vi "Process.vi"(8 "error in":errorcluster, 11 "SMO.ByRefWithEvents":refnum<class "SMO.ByRefWithEvents.lvclass">) -> (0 "error out":errorcluster, 3 "SMO.ByRefWithEvents out":refnum<class "SMO.ByRefWithEvents.lvclass">)   [LabVIEW 2013, in "SMO.ByRefWithEvents.lvclass"]
doc: "---------------------------------------------------------------\nJKI State Machine Objects™\nhttp://jki.net/state-machine-objects/\nCopyright (C) 2005-2015, JKI <info@jki.net>\nALL RIGHTS RESERVEDJKI State Machine Objects (SMO) 1.0.0.5\nJKI - JKI\nCopyright (c) 2016, JKI"
uses:
  SMO.ByRefWithEvents.lvclass
  <vilib>/JKI/JKI SMO/SMO/Typedefs/Parent Call--Enum.ctl
  <vilib>/JKI/JKI SMO/SMO/SMO.lvclass
panel:
  # "For instructions on how to use the JKI State Machine Objects, examples and video tutorials, visit:\nhttp://jki.net/state-machine-objects/\n\nJKI State Machine Objects™\nhttp://jki.net/state-machine-objects/\nCopyright (C) 2005-2015, JKI <info@jki.net>\nALL RIGHTS RESERVED"
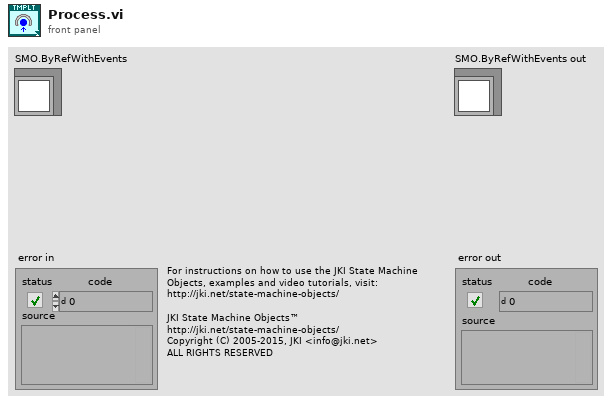
[diagram p1: front panel]
types:
  T1 = typedef "SMO.lvclass/Parent Call--Enum.ctl" = enum16{"Allows parent to run", "Does not request parent to run"}
  T2 = enum32{"invalid app kind", "Development System", "Run Time System", "Student Edition", "Embedded LabVIEW", "Evaluation", "Custom"}
  T3 = enum32{"Invalid", "Standard", "Closed", "Hidden", "Minimized", "Maximized"}
  T4 = enum32{"Bad", "Idle", "Run top level", "Running"}
  T5 = cluster{"Core":cluster{"Current VI Reference":refnum<vi>, "Close Panel on Exit?":bool, "error":errorcluster}, "Self Reference":refnum<class "SMO.ByRefWithEvents.lvclass">, "Your string data":string}
  T6 = cluster{"Current VI Reference":refnum<vi>, "Close Panel on Exit?":bool, "error":errorcluster}
  T7 = typedef "SMO.lvclass/Protected Events.ctl" = cluster{"StopProcesses":refnum<user-event>, "AbortProcesses":refnum<user-event>}
  T8 = typedef "SMO.ByRefWithEvents.lvclass/ProtectedEvents--Cluster.ctl" = cluster{"API_Template":refnum<user-event>}
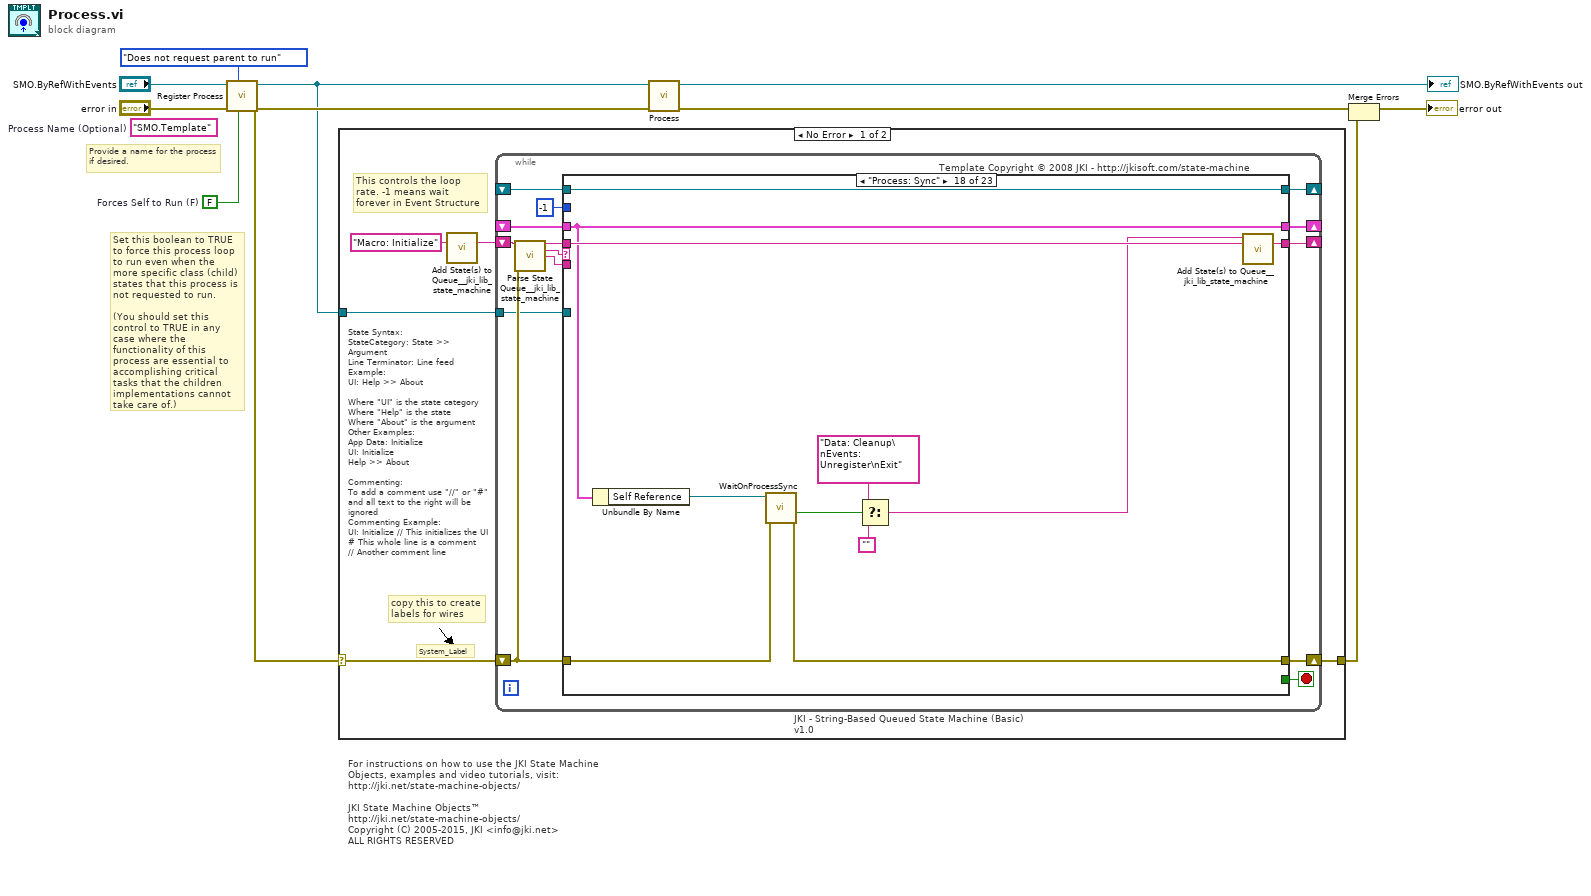
[diagram p0: block diagram]
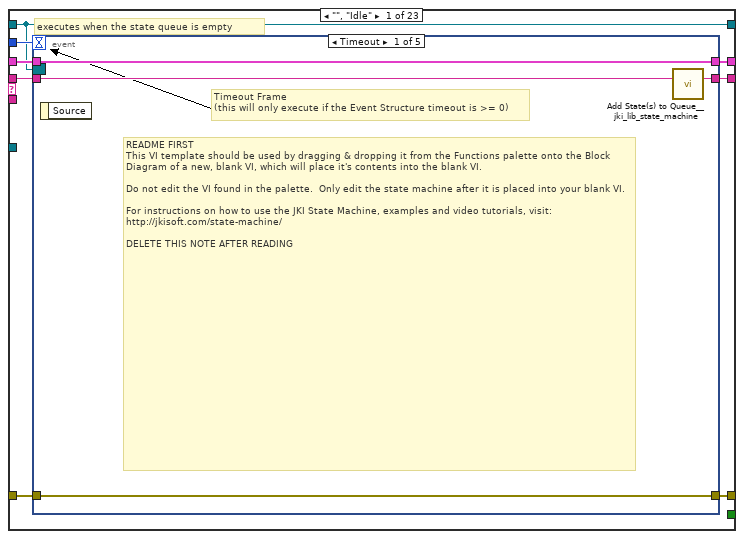
[diagram p2: hidden frame]
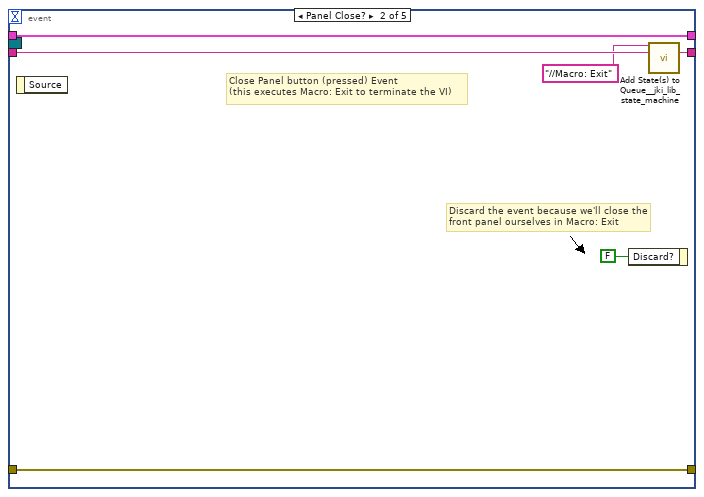
[diagram p3: hidden frame]
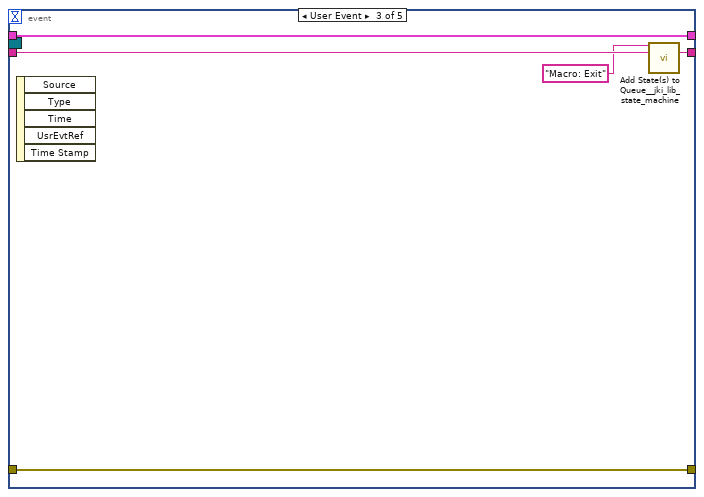
[diagram p4: hidden frame]
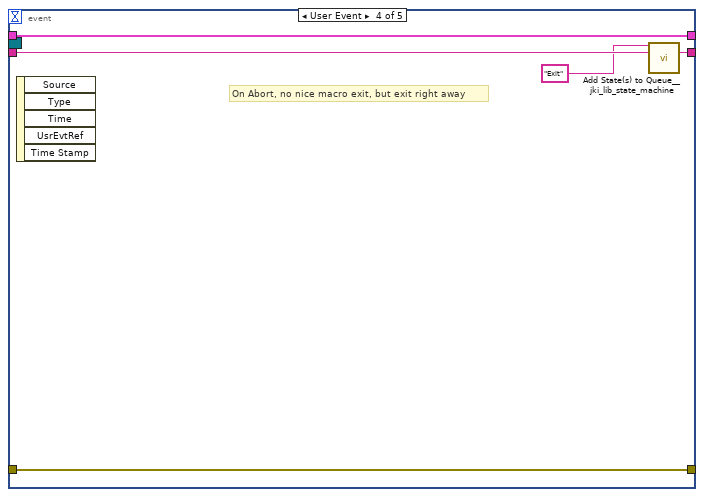
[diagram p5: hidden frame]
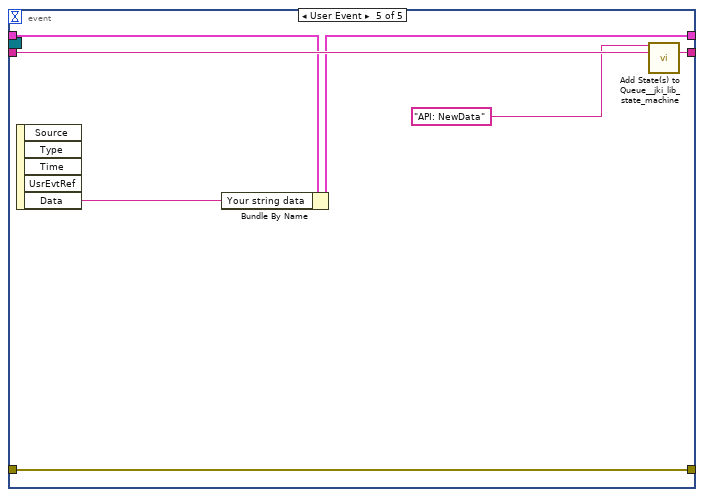
[diagram p6: hidden frame]
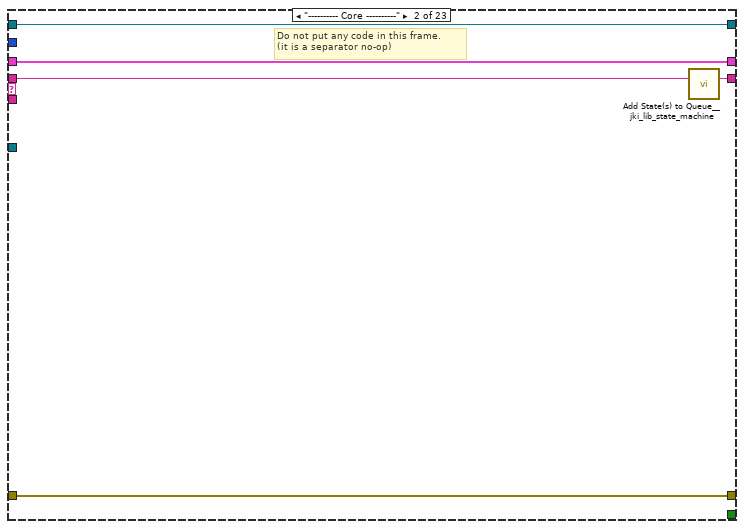
[diagram p7: hidden frame]
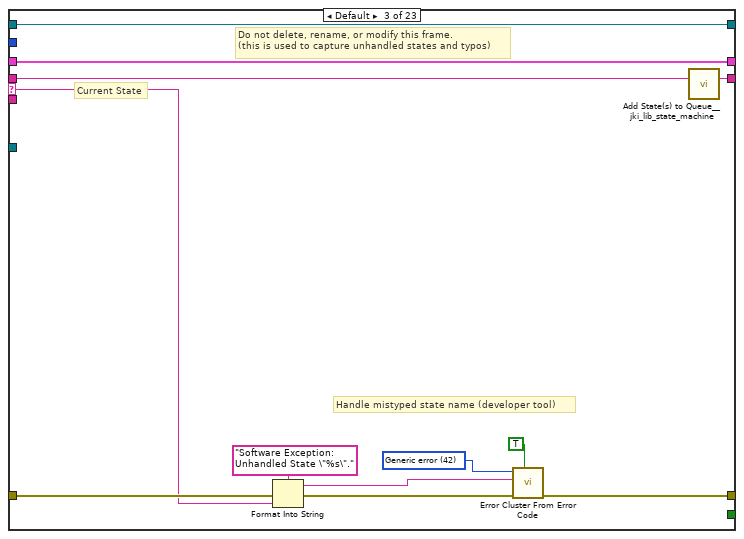
[diagram p8: hidden frame]
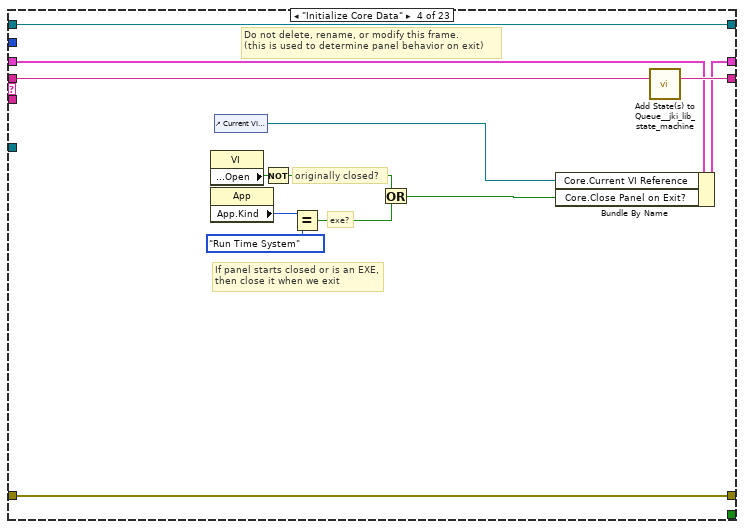
[diagram p9: hidden frame]
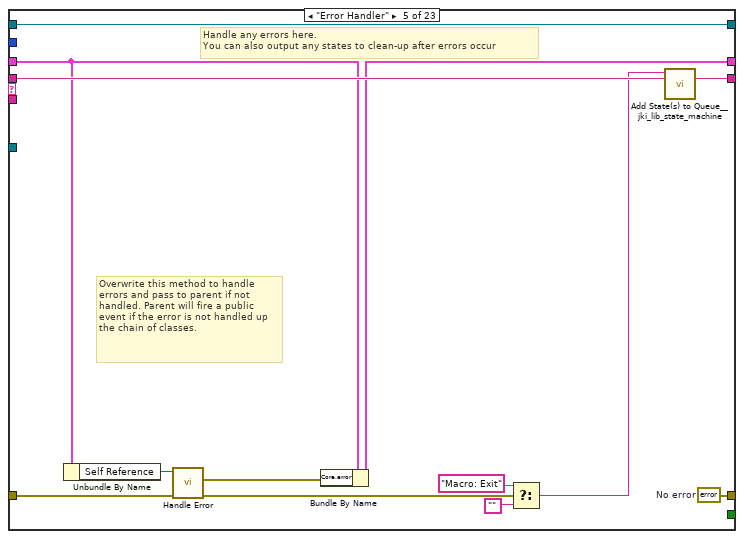
[diagram p10: hidden frame]
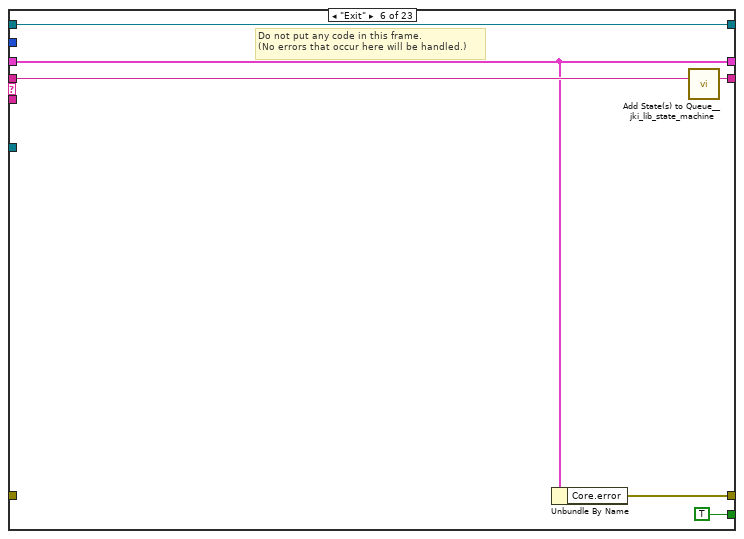
[diagram p11: hidden frame]
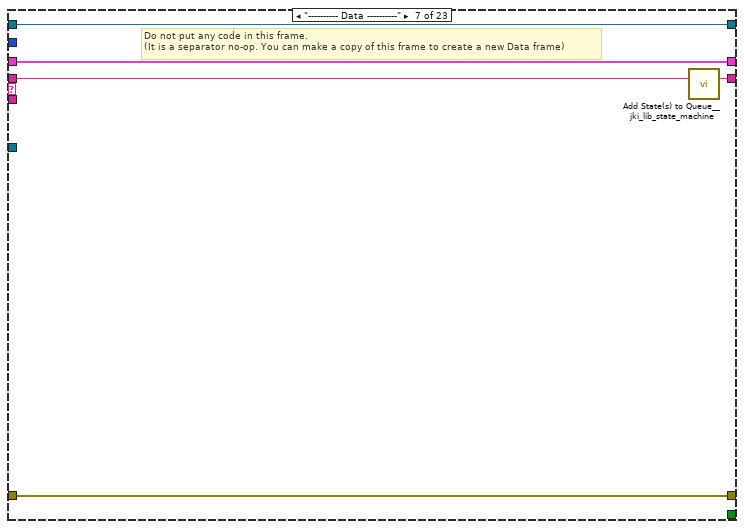
[diagram p12: hidden frame]
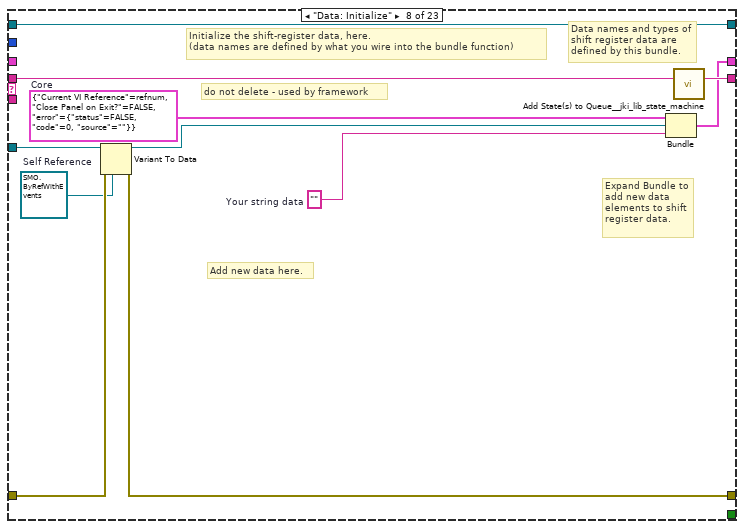
[diagram p13: hidden frame]
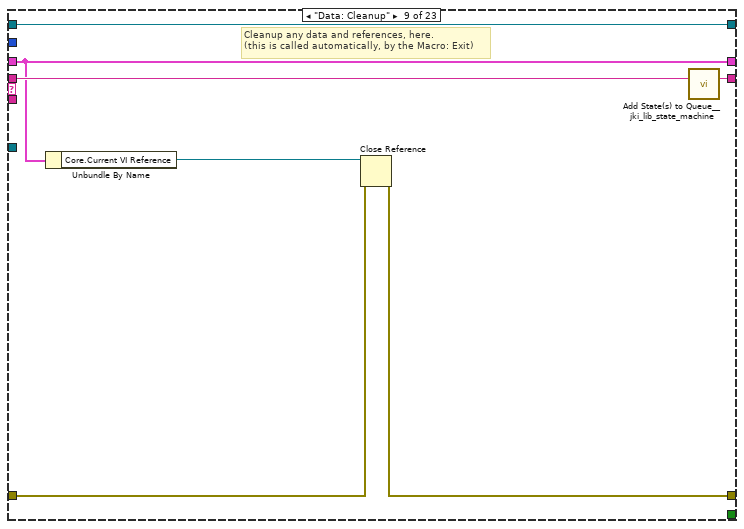
[diagram p14: hidden frame]
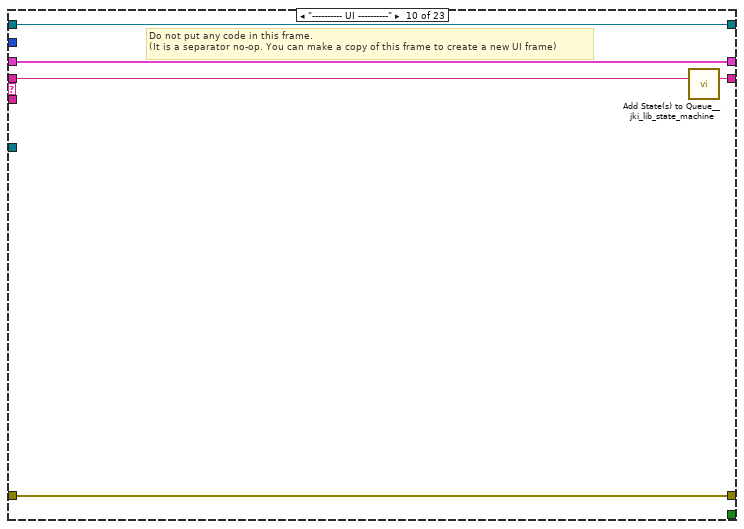
[diagram p15: hidden frame]
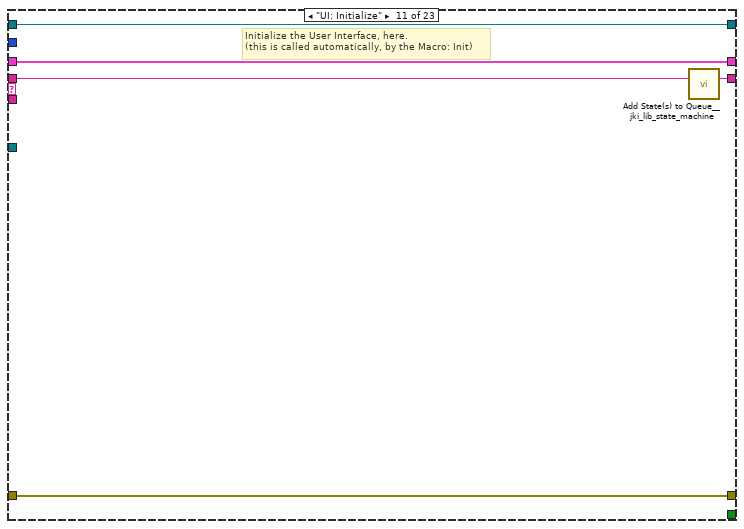
[diagram p16: hidden frame]
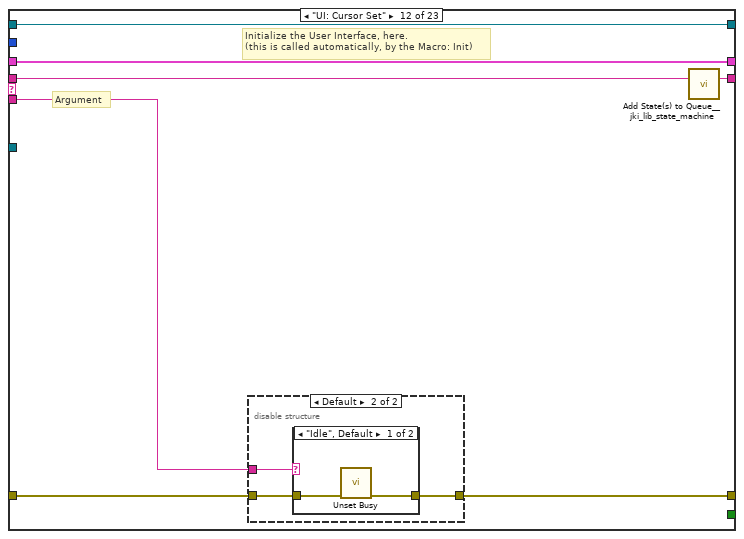
[diagram p17: hidden frame]
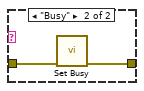
[diagram p19: hidden frame]
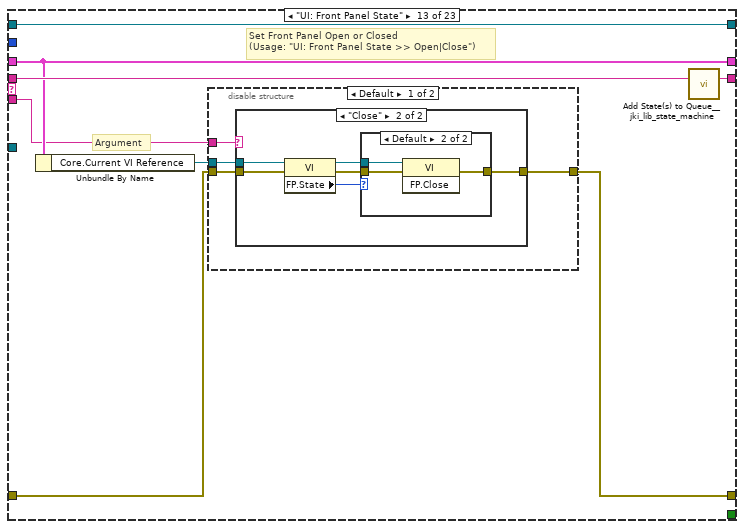
[diagram p20: hidden frame]
diagram:
  w1 = FALSE  # Forces Self to Run (F)
  (unwired) "SMO.Template"  # Process Name (Optional)
  # "Provide a name for the process\nif desired."
  # "Set this boolean to TRUE to force this process loop to run even when the more specific class (child) states that this process is not requested to run.\n\n(You should set this control to TRUE in any case where the functionality of this process are essential to accomplishing critical tasks that the children implementations cannot take care of.)"
  # "For instructions on how to use the JKI State Machine Objects, examples and video tutorials, visit:\nhttp://jki.net/state-machine-objects/\n\nJKI State Machine Objects™\nhttp://jki.net/state-machine-objects/\nCopyright (C) 2005-2015, JKI <info@jki.net>\nALL RIGHTS RESERVED"
  n1 = call <vilib>:"Register Process.vi"("Forces Self to Run (F)"=w1, "Parent Call"=Parent_Call--Enum."Does not request parent to run", "error in (no error)"="error in", "SMO"="SMO.ByRefWithEvents") -> ("error out"=w7:errorcluster, "SMO out"=w6:refnum<class "SMO.ByRefWithEvents.lvclass">)  [unwired: 6 in]
  n2 = case shown="No Error" w7 {
    selector: w7 -> [w12 w295]
    tunnel: w6 -> [w13 _]
    tunnel: [w11 w295] -> w3
    frame No Error {
      # "State Syntax:\nStateCategory: State >> Argument\nLine Terminator: Line feed\nExample:\nUI: Help >> About\n\nWhere \"UI\" is the state category\nWhere \"Help\" is the state\nWhere \"About\" is the argument\nOther Examples:\nApp Data: Initialize\nUI: Initialize\nHelp >> About\n\nCommenting:\nTo add a comment use \"//\" or \"#\" and all text to the right will be ignored\nCommenting Example:\nUI: Initialize // This initializes the UI\n# This whole line is a comment\n// Another comment line"
      # "copy this to create labels for wires"
      # "This controls the loop rate. -1 means wait forever in Event Structure"
      # "System_Label"
      n3 = call <vilib>:"Add State(s) to Queue__jki_lib_state_machine.vi"("State(s) in (\"\")"="Macro: Initialize") -> ("States Out"=w15:string)  [unwired: 14 in]
      n4 = while "JKI - String-Based Queued State Machine (Basic) v1.0" {
        shift-right: [w22] -> _
        shift-left: _ -> [w21]
        shift-right: [w25] -> w11
        shift-left: w12 -> [w19]
        shift-right: [w24] -> _
        shift-left: w15 -> [w26]
        tunnel: w13 -> [w18]
        shift-right: [w17] -> _
        shift-left: _ -> [w16]
        stop <- w23 stop-if-true
        # "Template Copyright © 2008 JKI - http://jkisoft.com/state-machine"
        n5 = call <vilib>:"Parse State Queue__jki_lib_state_machine.vi"("State Queue"=w26, "Error In (no error)"=w19) -> ("Remaining States"=w28:string, "Current State"=w29:string, "Arguments"=w27:string)  [unwired: 11 in]
        n6 = case shown="\"Process: Sync\"" w29 {
          selector: w29 -> [_ _ w71 _ _ _ _ _ _ _ _ _ _ _ _ _ _ _ _ _ _ _ _]
          tunnel: w28 -> [w37 w69 w75 w94 w107 w113 w118 w129 w136 w141 w146 w153 w169 w201 w215 w229 w234 w245 w250 w264 w281 w286 w294]
          tunnel: w27 -> [_ _ _ _ _ _ _ _ _ _ _ w147 w163 _ _ _ _ _ _ _ _ _ _]
          tunnel: w21 -> [w35 w66 w73 w85 w96 w109 w115 _ w131 w138 w144 w151 w165 w198 w211 w220 w231 w242 w247 w262 w279 w284 w291]
          tunnel: [w34 w67 w77 w91 w98 w108 w116 w124 w132 w139 w143 w148 w166 w199 w213 w227 w232 w236 w248 w260 w276 w282 w287] -> w25
          tunnel: w19 -> [w33 w67 w76 w91 w103 _ w116 w125 w133 w139 w143 w149 w167 w199 w213 w227 w232 w237 w248 w261 w277 w282 w288]
          tunnel: [w36 w68 w74 w93 w106 w112 w117 w128 w135 w140 w145 w152 w168 w200 w214 w228 w233 w244 w249 w263 w280 w285 w293] -> w24
          tunnel: [_ _ _ _ _ TRUE _ _ _ _ _ _ _ _ _ _ _ _ _ _ _ _ _] -> w23
          tunnel: [w32 w66 w73 w92 w95 w109 w115 w127 w131 w138 w144 w151 w165 w198 w211 w220 w231 w242 w247 w262 w279 w284 w291] -> w22
          tunnel: -1 ("Timeout") -> [w31 _ _ _ _ _ _ _ _ _ _ _ _ _ _ _ _ _ _ _ _ _ _]
          tunnel: w18 -> [_ _ _ _ _ _ _ w122 _ _ _ _ _ _ _ _ _ _ _ _ _ _ _]
          tunnel: [w30 w65 w70 w82 w105 w110 w114 w120 w130 w137 w142 w150 w162 w197 w212 w221 w230 w243 w246 w259 w278 w283 w292] -> w17
          tunnel: w16 -> [w30 w65 w70 w82 w105 w110 w114 w120 w130 w137 w142 w150 w162 w197 w212 w221 w230 w243 w246 w251 w278 w283 w292]
          frame "", "Idle" {
            # "executes when the state queue is empty"
            n7 = event shown="[0] Timeout" {
              selector: w30 -> [_ _ _ _ _]
              dyn-events: _ -> [_ _ _ _ _]
              timeout: w31 -> [_ _ _ _ _]
              tunnel: w37 -> [w41 w47 w52 w57 w64]
              tunnel: [w40 w46 w51 w56 w63] -> w36
              tunnel: w35 -> [w38 w44 w49 w54 w60]
              tunnel: [w39 w45 w50 w55 w62] -> w34
              tunnel: w33 -> [w39 w45 w50 w55 w62]
              tunnel: [w38 w44 w49 w54 w59] -> w32
              event Timeout {
                # "README FIRST\nThis VI template should be used by dragging & dropping it from the Functions palette onto the Block Diagram of a new, blank VI, which will place it's contents into the blank VI.\n\nDo not edit the VI found in the palette.  Only edit the state machine after it is placed into your blank VI.\n\nFor instructions on how to use the JKI State Machine, examples and video tutorials, visit:\nhttp://jkisoft.com/state-machine/\n\nDELETE THIS NOTE AFTER READING"
                # "Timeout Frame\n(this will only execute if the Event Structure timeout is >= 0)"
                n8 = event-data() -> ()  [unwired: 1 in, 1 out]
                n9 = call <vilib>:"Add State(s) to Queue__jki_lib_state_machine.vi"("State(s) in (\"\")"=w41) -> ("States Out"=w40:string)  [unwired: 14 in]
              }
              event Panel Close? {
                # "Discard the event because we'll close the front panel ourselves in Macro: Exit"
                # "Close Panel button (pressed) Event\n(this executes Macro: Exit to terminate the VI)"
                n10 = event-data() -> ()  [unwired: 1 in, 1 out]
                n11 = event-data("Discard?"=FALSE) -> ()  [unwired: 1 in, 1 out]
                n12 = call <vilib>:"Add State(s) to Queue__jki_lib_state_machine.vi"("State(s) in Front (\"\")"="//Macro: Exit", "State(s) in (\"\")"=w47) -> ("States Out"=w46:string)  [unwired: 13 in]
              }
              event User Event {
                n13 = event-data() -> ()  [unwired: 1 in, 5 out]
                n14 = call <vilib>:"Add State(s) to Queue__jki_lib_state_machine.vi"("State(s) in Front (\"\")"="Macro: Exit", "State(s) in (\"\")"=w52) -> ("States Out"=w51:string)  [unwired: 13 in]
              }
              event User Event {
                # "On Abort, no nice macro exit, but exit right away"
                n15 = event-data() -> ()  [unwired: 1 in, 5 out]
                n16 = call <vilib>:"Add State(s) to Queue__jki_lib_state_machine.vi"("State(s) in Front (\"\")"="Exit", "State(s) in (\"\")"=w57) -> ("States Out"=w56:string)  [unwired: 13 in]
              }
              event User Event {
                n17 = event-data() -> ("Data"=w61:string)  [unwired: 1 in, 4 out]
                n18 = Bundle By Name(cluster=w60, "Your string data"=w61) -> (w59:T5)
                n19 = call <vilib>:"Add State(s) to Queue__jki_lib_state_machine.vi"("State(s) in Front (\"\")"="API: NewData", "State(s) in (\"\")"=w64) -> ("States Out"=w63:string)  [unwired: 13 in]
              }
            }
          }
          frame "---------- Core ----------" {
            # "Do not put any code in this frame.\n(it is a separator no-op)"
            n20 = call <vilib>:"Add State(s) to Queue__jki_lib_state_machine.vi"("State(s) in (\"\")"=w69) -> ("States Out"=w68:string)  [unwired: 14 in]
          }
          frame Default {
            w80 = 42 items=["No error", "Argument error", "Memory is full", "Out of zone", "End of file", "File already open", "Generic file I/O error", "File not found", "File permission error", "Disk is full", "Duplicate path", "Too many files open", "System feature not enabled", "Resource file not found", "Cannot add resource", "Resource not found", "Image not found", "Image memory error", "Pen does not exist", "Config type invalid", "Config token not found", "Config parse error", "Config memory error", "Bad external code format", "Bad external code offset", "External code not present", "Null window", "Destroy window error", "Null menu", "Print aborted", "Bad print record", "Print driver error", "Windows error during printing", "Memory error during printing", "Print dialog error", "Generic print error", "Invalid device refnum", "Device not found", "Device parameter error", "Device unit error", "Cannot open device", "Device call aborted", "Generic error", "Cancelled by user", "Object ID too low", "Object ID too high", "Object not in heap", "Unknown heap", "Unknown object (invalid DefProc)", "Unknown object (DefProc not in table)", "Message out of range", "Invalid (null) method", "Unknown message", "Manager call not supported", "Bad address", "Network operation in progress", "Network operation timed out", "Connection is busy", "Network attribute not supported", "Network error", "Address in use", "System out of memory", "Connection aborted", "Connection refused", "Not connected", "Already connected", "Connection closed", "Initialization error (interapplication manager)", "Bad occurrence", "Wait on unbound occurrence handler", "Occurrence queue overflow", "Datalog type conflict", "Unused", "Unrecognized type (interapplication manager)", "Memory corrupt", "Failed to make temporary DLL", "Old CIN version", "Drag socket not found", "Failed to load drop-object", "Failed to register OLE object", "Failed to release OLE object", "Format specifier type mismatch", "Unknown format specifier", "Too few format specifiers", "Too many format specifiers", "Scan failed", "Newer CIN version", "Error converting to variant", "Runtime menu error", "Password tampered", "Variant attribute not found", "Incompatible variant data type", "Event data is not available", "Event Store is not present", "Occurrence is not found", "Event Queue is not created", "Event info is not available", "Refnum passed is NULL", "Error retrieving Class GUID", "Error retrieving CoClass GUID", "Error retrieving TypeLib GUID.", "Bad built application magic bytes.", "Specific driver is different from the specific driver associated with the Logical Name.", "There is no session opened to the class driver.", "Max Error", "MAX - Error with config objects", "MAX - Error loading configuration", "MAX - Group not supported"]
            # "Current State"
            # "Do not delete, rename, or modify this frame.\n(this is used to capture unhandled states and typos)"
            # "Handle mistyped state name (developer tool)"
            n21 = Format Into String(format string="Software Exception: Unhandled State \"%s\"." ("message"), error in=w76, w71) -> (resulting string=w79:string, error out=w78:errorcluster)  [unwired: 1 in]
            n22 = call <vilib>:"Error Cluster From Error Code.vi"("show call chain? (False)"=TRUE, "error in (no error)"=w78, "error message (\"\")"=w79, "error code (0)"=w80) -> ("error out"=w77:errorcluster)  [unwired: 5 in]
            n23 = call <vilib>:"Add State(s) to Queue__jki_lib_state_machine.vi"("State(s) in (\"\")"=w75) -> ("States Out"=w74:string)  [unwired: 14 in]
          }
          frame "Initialize Core Data" {
            # "Do not delete, rename, or modify this frame.\n(this is used to determine panel behavior on exit)"
            # "originally closed?"
            # "exe?"
            # "If panel starts closed or is an EXE, then close it when we exit"
            n24 = property class="VI"() -> ("Front Panel.Open"=w90:bool)  [unwired: 2 in, 2 out]
            n25 = property class="App"() -> ("App.Kind"=w89:T2)  [unwired: 2 in, 2 out]
            n26 = control-ref of="Current VI Reference"() -> (w83:refnum<vi>)
            n27 = Not(x=w90) -> (.not. x?=w87:bool)
            n28 = Equal?(x=w89, y=T2."Run Time System" ("Application:Kind")) -> (x = y?=w86:bool)
            n29 = Or(x=w87, y=w86) -> (x .or. y?=w84:bool)
            n30 = Bundle By Name(cluster=w85, "Core.Current VI Reference"=w83, "Core.Close Panel on Exit?"=w84) -> (w92:T5)
            n31 = call <vilib>:"Add State(s) to Queue__jki_lib_state_machine.vi"("State(s) in (\"\")"=w94) -> ("States Out"=w93:string)  [unwired: 14 in]
          }
          frame "Error Handler" {
            w98 = errorcluster {"status"=FALSE, "code"=0, "source"=""}  # No error
            # "Overwrite this method to handle errors and pass to parent if not handled. Parent will fire a public event if the error is not handled up the chain of classes."
            # "Handle any errors here.\nYou can also output any states to clean-up after errors occur"
            n32 = Unbundle By Name(w96) -> ("Self Reference"=w104:refnum<class "SMO.ByRefWithEvents.lvclass">)
            n33 = call-dynamic "Handle Error.vi"("error in"=w103, "SMO"=w104) -> ("handling error"=w99:errorcluster, "Unhandled error"=w97:errorcluster)  [unwired: 7 in, 1 out]
            n34 = Bundle By Name(cluster=w96, "Core.error"=w97) -> (w95:T5)
            n35 = Select(t="Macro: Exit", s=w99, f="") -> (s? t:f=w100:string)
            n36 = call <vilib>:"Add State(s) to Queue__jki_lib_state_machine.vi"("State(s) in Front (\"\")"=w100, "State(s) in (\"\")"=w107) -> ("States Out"=w106:string)  [unwired: 13 in]
          }
          frame "Exit" {
            # "Do not put any code in this frame.\n(No errors that occur here will be handled.)"
            n37 = Unbundle By Name(w109) -> ("Core.error"=w108:errorcluster)
            n38 = call <vilib>:"Add State(s) to Queue__jki_lib_state_machine.vi"("State(s) in (\"\")"=w113) -> ("States Out"=w112:string)  [unwired: 14 in]
          }
          frame "---------- Data ----------" {
            # "Do not put any code in this frame.\n(It is a separator no-op. You can make a copy of this frame to create a new Data frame)"
            n39 = call <vilib>:"Add State(s) to Queue__jki_lib_state_machine.vi"("State(s) in (\"\")"=w118) -> ("States Out"=w117:string)  [unwired: 14 in]
          }
          frame "Data: Initialize" {
            w119 = T6 {"Current VI Reference"=refnum, "Close Panel on Exit?"=FALSE, "error"={"status"=FALSE, "code"=0, "source"=""}}  # Core
            w123 = refnum<class "SMO.ByRefWithEvents.lvclass"> refnum  # Self Reference
            w126 = ""  # Your string data
            # "do not delete - used by framework"
            # "Expand Bundle to add new data elements to shift register data."
            # "Add new data here."
            # "Data names and types of shift register data are defined by this bundle."
            # "Initialize the shift-register data, here.\n(data names are defined by what you wire into the bundle function)"
            n40 = Variant To Data(error in=w125, type=w123, Variant=w122) -> (data=w121:refnum<class "SMO.ByRefWithEvents.lvclass">, error out=w124:errorcluster)
            n41 = Bundle("Core"=w119, "Self Reference"=w121, "Your string data"=w126) -> (w127:T5)  [unwired: 1 in]
            n42 = call <vilib>:"Add State(s) to Queue__jki_lib_state_machine.vi"("State(s) in (\"\")"=w129) -> ("States Out"=w128:string)  [unwired: 14 in]
          }
          frame "Data: Cleanup" {
            # "Cleanup any data and references, here.\n(this is called automatically, by the Macro: Exit)"
            n43 = Unbundle By Name(w131) -> ("Core.Current VI Reference"=w134:refnum<vi>)
            n44 = Close Reference(reference=w134, error in (no error)=w133) -> (error out=w132:errorcluster)
            n45 = call <vilib>:"Add State(s) to Queue__jki_lib_state_machine.vi"("State(s) in (\"\")"=w136) -> ("States Out"=w135:string)  [unwired: 14 in]
          }
          frame "---------- UI ----------" {
            # "Do not put any code in this frame.\n(It is a separator no-op. You can make a copy of this frame to create a new UI frame)"
            n46 = call <vilib>:"Add State(s) to Queue__jki_lib_state_machine.vi"("State(s) in (\"\")"=w141) -> ("States Out"=w140:string)  [unwired: 14 in]
          }
          frame "UI: Initialize" {
            # "Initialize the User Interface, here.\n(this is called automatically, by the Macro: Init)"
            n47 = call <vilib>:"Add State(s) to Queue__jki_lib_state_machine.vi"("State(s) in (\"\")"=w146) -> ("States Out"=w145:string)  [unwired: 14 in]
          }
          frame "UI: Cursor Set" {
            # "Argument"
            # "Initialize the User Interface, here.\n(this is called automatically, by the Macro: Init)"
            n48 = disable-structure shown="Default" {
              disable-tunnel: w149 -> [w154 w157]
              disable-tunnel: [w154 w156] -> w148
              disable-tunnel: w147 -> [_ w155]
              frame condition #0 {
              }
              frame condition #1 (active) {
                n49 = case shown="\"Idle\", Default" w155 {
                  tunnel: w157 -> [w159 w161]
                  tunnel: [w158 w160] -> w156
                  frame "Idle", Default {
                    n50 = call <vilib>:"Unset Busy.vi"("error in (no error)"=w159) -> ("error out"=w158:errorcluster)  [unwired: 10 in]
                  }
                  frame "Busy" {
                    n51 = call <vilib>:"Set Busy.vi"("error in (no error)"=w161) -> ("error out"=w160:errorcluster)  [unwired: 9 in, 1 out]
                  }
                }
              }
            }
            n52 = call <vilib>:"Add State(s) to Queue__jki_lib_state_machine.vi"("State(s) in (\"\")"=w153) -> ("States Out"=w152:string)  [unwired: 14 in]
          }
          frame "UI: Front Panel State" {
            # "Argument"
            # "Set Front Panel Open or Closed\n(Usage: \"UI: Front Panel State >> Open|Close\")"
            n53 = Unbundle By Name(w165) -> ("Core.Current VI Reference"=w164:refnum<vi>)
            n54 = disable-structure shown="Default" {
              disable-tunnel: w167 -> [w173 w196]
              disable-tunnel: [w172 w196] -> w166
              disable-tunnel: w164 -> [w171 _]
              disable-tunnel: w163 -> [w170 _]
              frame condition #0 (active) {
                n55 = case shown="\"Close\"" w170 {
                  tunnel: w173 -> [w177 w190]
                  tunnel: [w179 w191] -> w172
                  tunnel: w171 -> [w178 w188]
                  frame "Open", Default {
                    n56 = property class="VI"(reference=w178, error in=w177) -> (reference out=w175:refnum<vi>, error out=w176:errorcluster, "FP.State"=w174:T3)
                    n57 = case shown="\"Closed\"" w174 {
                      tunnel: [w182 w185] -> w179
                      tunnel: w176 -> [w181 w185]
                      tunnel: w175 -> [w180 _]
                      frame "Closed" {
                        n58 = invoke class="VI" method="FP.Open"(reference=w180, error in=w181, "Activate"=TRUE, "State"=T3."Standard") -> (error out=w182:errorcluster)  [unwired: 1 in, 4 out]
                      }
                      frame Default {
                      }
                    }
                  }
                  frame "Close" {
                    n59 = property class="VI"(reference=w188, error in=w190) -> (reference out=w187:refnum<vi>, error out=w189:errorcluster, "FP.State"=w186:T3)
                    n60 = case shown="Default" w186 {
                      tunnel: [w192 w195] -> w191
                      tunnel: w189 -> [w192 w194]
                      tunnel: w187 -> [_ w193]
                      frame "Invalid", "Closed" {
                      }
                      frame Default {
                        n61 = invoke class="VI" method="FP.Close"(reference=w193, error in=w194) -> (error out=w195:errorcluster)  [unwired: 1 in, 2 out]
                      }
                    }
                  }
                }
              }
              frame condition #1 {
              }
            }
            n62 = call <vilib>:"Add State(s) to Queue__jki_lib_state_machine.vi"("State(s) in (\"\")"=w169) -> ("States Out"=w168:string)  [unwired: 14 in]
          }
          frame "---------- Macro ----------" {
            # "Do not put any code in this frame.\n(It is a separator no-op. You can make a copy of this frame to create a new Macro frame)"
            n63 = call <vilib>:"Add State(s) to Queue__jki_lib_state_machine.vi"("State(s) in (\"\")"=w201) -> ("States Out"=w200:string)  [unwired: 14 in]
          }
          frame "Macro: Initialize" {
            w206 = "//UI: Initialize\n//UI: Front Panel State >> Open"  # //UI: Initialize //UI: Front Panel State >> Open
            w202 = "Process: Sync"
            # "Initialization Macro\n(This is called once, when the VI starts)"
            n64 = control-ref of="This VI"() -> (w204:refnum<vi>)
            n65 = property class="VI"(reference=w204) -> ("Exec.State"=w203:T4)  [unwired: 1 in, 2 out]
            n66 = Equal?(x=w203, y=T4."Run top level") -> (x = y?=w209:bool)
            n67 = Select(t=w202, s=w209, f="") -> ()  [unwired: 1 out]
            n68 = call <vilib>:"Add State(s) to Queue__jki_lib_state_machine.vi"("State(s) in Front (\"\")"="Data: Initialize\nInitialize Core Data\nEvents: Register", "State(s) in (\"\")"=w202, "State(s) at Back (\"\")"=w206) -> ("States Out"=w205:string)  [unwired: 12 in]
            n69 = call <vilib>:"Add State(s) to Queue__jki_lib_state_machine.vi"("State(s) in Front (\"\")"=w205, "State(s) in (\"\")"=w215) -> ("States Out"=w214:string)  [unwired: 13 in]
          }
          frame "Macro: Exit" {
            # "Exit Macro\n(This is called once, when the VI exits)"
            n70 = Unbundle By Name(w220) -> ("Core.Close Panel on Exit?"=w226:bool)
            n71 = Select(t="UI: Front Panel State >> Close", s=w226, f="") -> (s? t:f=w223:string)
            n72 = call <vilib>:"Add State(s) to Queue__jki_lib_state_machine.vi"("State(s) in Front (\"\")"="Data: Cleanup\nEvents: Unregister", "State(s) in (\"\")"="Process: Sync", "State(s) at Back (\"\")"="Exit") -> ("States Out"=w217:string)  [unwired: 12 in]
            n73 = call <vilib>:"Add State(s) to Queue__jki_lib_state_machine.vi"("State(s) in (\"\")"=w223, "State(s) at Back (\"\")"=w217) -> ("States Out"=w222:string)  [unwired: 13 in]
            n74 = call <vilib>:"Add State(s) to Queue__jki_lib_state_machine.vi"("State(s) in Front (\"\")"=w222, "State(s) in (\"\")"=w229) -> ("States Out"=w228:string)  [unwired: 13 in]
          }
          frame "---------- Process ----------" {
            # "Template Separator\n(You can make a copy of, or modify, this frame)"
            n75 = call <vilib>:"Add State(s) to Queue__jki_lib_state_machine.vi"("State(s) in (\"\")"=w234) -> ("States Out"=w233:string)  [unwired: 14 in]
          }
          frame "Process: Sync" {
            n76 = Unbundle By Name(w242) -> ("Self Reference"=w238:refnum<class "SMO.ByRefWithEvents.lvclass">)
            n77 = call <vilib>:"WaitOnProcessSync.vi"("error in (no error)"=w237, "SMO"=w238) -> ("error out"=w236:errorcluster, "Don't run?"=w241:bool)  [unwired: 7 in, 1 out]
            n78 = Select(t="Data: Cleanup\nEvents: Unregister\nExit", s=w241, f="") -> (s? t:f=w235:string)
            n79 = call <vilib>:"Add State(s) to Queue__jki_lib_state_machine.vi"("State(s) in Front (\"\")"=w235, "State(s) in (\"\")"=w245) -> ("States Out"=w244:string)  [unwired: 13 in]
          }
          frame "---------- Events ----------" {
            # "Template Separator\n(You can make a copy of, or modify, this frame)"
            n80 = call <vilib>:"Add State(s) to Queue__jki_lib_state_machine.vi"("State(s) in (\"\")"=w250) -> ("States Out"=w249:string)  [unwired: 14 in]
          }
          frame "Events: Register" {
            # "Self Events (API Calls)"
            # "Base Class Protected Events"
            n81 = Unbundle By Name(w262) -> ("Self Reference"=w253:refnum<class "SMO.ByRefWithEvents.lvclass">)
            n82 = call <vilib>:"GetProtectedEvents.vi"("error in (no error)"=w261, "SMO"=w253) -> ("error out"=w256:errorcluster, "SMO Protected Events"=w258:T7, "SMO out"=w257:refnum<class "SMO.ByRefWithEvents.lvclass">)  [unwired: 7 in]
            n83 = call "SMO.ByRefWithEvents.GetProtectedEvents.vi"("error in (no error)"=w256, "SMO.ByRefWithEvents"=w257) -> ("error out"=w255:errorcluster, "Protected Events"=w254:T8)  [unwired: 7 in, 1 out]
            n84 = Not A Number/Path/Refnum?(number/path/refnum=w251) -> (NaN/Path/Refnum?=w252:bool)
            n85 = case shown="True" w252 {
              tunnel: [w269 w275] -> w260
              tunnel: [w268 w274] -> w259
              tunnel: w258 -> [w267 w273]
              tunnel: w255 -> [w266 w272]
              tunnel: w254 -> [w265 w271]
              tunnel: w251 -> [_ w270]
              frame True {
                # "Expand to add\nmore events"
                n86 = register-events(error in=w266, w267, w265) -> (reference out=w268:refnum<event-registration>, error out=w269:errorcluster)  [unwired: 1 in]
              }
              frame False {
                n87 = register-events(reference=w270, error in=w272, w273, w271) -> (reference out=w274:refnum<event-registration>, error out=w275:errorcluster)
              }
            }
            n88 = call <vilib>:"Add State(s) to Queue__jki_lib_state_machine.vi"("State(s) in (\"\")"=w264) -> ("States Out"=w263:string)  [unwired: 14 in]
          }
          frame "Events: Unregister" {
            n89 = Unregister For Events(event registration refnum=w278, error in=w277) -> (error out=w276:errorcluster)
            n90 = call <vilib>:"Add State(s) to Queue__jki_lib_state_machine.vi"("State(s) in (\"\")"=w281) -> ("States Out"=w280:string)  [unwired: 14 in]
          }
          frame "---------- API ----------" {
            n91 = call <vilib>:"Add State(s) to Queue__jki_lib_state_machine.vi"("State(s) in (\"\")"=w286) -> ("States Out"=w285:string)  [unwired: 14 in]
          }
          frame "API: NewData" {
            n92 = Unbundle By Name(w291) -> ("Self Reference"=w290:refnum<class "SMO.ByRefWithEvents.lvclass">, "Your string data"=w289:string)
            n93 = call "SMO.ByRefWithEvents.SetData.vi"("error in (no error)"=w288, "Data In"=w289, "SMO.ByRefWithEvents"=w290) -> ("error out"=w287:errorcluster)  [unwired: 7 in, 1 out]
            n94 = call <vilib>:"Add State(s) to Queue__jki_lib_state_machine.vi"("State(s) in (\"\")"=w294) -> ("States Out"=w293:string)  [unwired: 14 in]
          }
        }
      }
    }
    frame Error {
    }
  }
  n95 = call-parent "Process.vi"("error in"=w7, "SMO"=w6) -> ("error out"=w4:errorcluster, "SMO out"=→"SMO.ByRefWithEvents out":refnum<class "SMO.ByRefWithEvents.lvclass">)  [unwired: 8 in]
  n96 = Merge Errors(w4, w3) -> (→"error out":errorcluster)
